vi "Actor Core.vi"(8 "error in":errorcluster, 11 "Flex UI (Actor) in":refnum<class "Flex UI (Actor).lvclass">) -> (0 "error out":errorcluster, 3 "Actor out":refnum<class "Actor.lvclass">)   [LabVIEW 2014, in "Flex UI (Parent Actor).lvlib" / "Flex UI (Actor).lvclass"]
doc: "(<B>Filename</B>: Actor Framework.lvlib:Actor.lvclass:Actor Core.vi)\n\nReceives messages to the actor, reacts to them, and initiates any error handling that may shut the actor down.\n\nDescendant classes may override this VI to append parallel tasks for the actor to complete while it handles messages. Overrides use the Call Parent Method node."
uses:
  Flex UI (Actor).lvclass
  <vilib>/ActorFramework/Actor/Actor.lvclass
  <vilib>/East West Architects/Parent Actor Template/_Parent Actor Template.lvclass
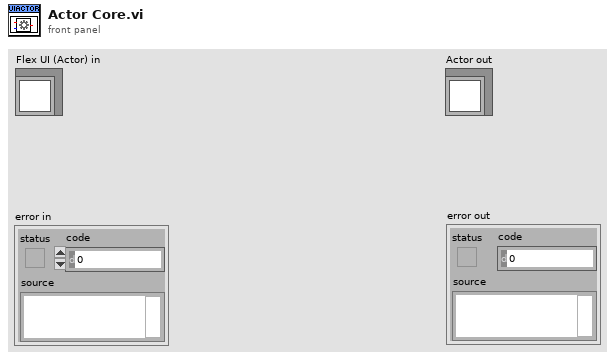
[diagram p1: front panel]
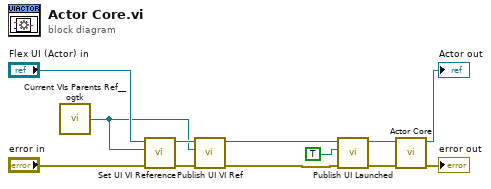
[diagram p0: block diagram]
diagram:
  n1 = call <userlib>:"Current VIs Parents Ref__ogtk.vi"() -> ("Calling VI's Reference"=w2:refnum<vi>)  [unwired: 2 in]
  n2 = call-dynamic "Set UI VI Reference.vi"("error in (no error)"="error in", "UI VI Reference (caller)"=w2, "Flex UI (Actor) in"="Flex UI (Actor) in") -> ("error out"=w7:errorcluster, "Flex UI (Actor) out"=w3:refnum<class "Flex UI (Actor).lvclass">)  [unwired: 7 in]
  n3 = call-dynamic "Publish UI VI Ref.vi"("error in (no error)"=w7, "VI Ref"=w2, "Flex UI (Actor) in"=w3) -> ("error out"=w4:errorcluster, "Flex UI (Actor) out"=w1:refnum<class "Flex UI (Actor).lvclass">)  [unwired: 7 in]
  n4 = call "Publish UI Launched.vi"("error in"=w4, "Launched"=TRUE, "Flex UI (Actor) in"=w1) -> ("error out"=w8:errorcluster, "Flex UI (Actor) out"=w5:refnum<class "Flex UI (Actor).lvclass">)  [unwired: 7 in]
  n5 = call-parent "Actor Core.vi"("error in"=w8, "_Parent Actor Template in"=w5) -> ("error out"=→"error out":errorcluster, "Actor out"=→"Actor out":refnum<class "Actor.lvclass">)  [unwired: 8 in]
